vi "About Design.vi"(8 "error in":errorcluster, 10 "Mathcad Output":T1, 11 "DesignRequest":T2) -> (0 "error out":errorcluster)   [LabVIEW 2012, in "Design Server.lvlib"]
uses:
  Design Server.lvlib
  Design Request.ctl
  Variable cluster.ctl
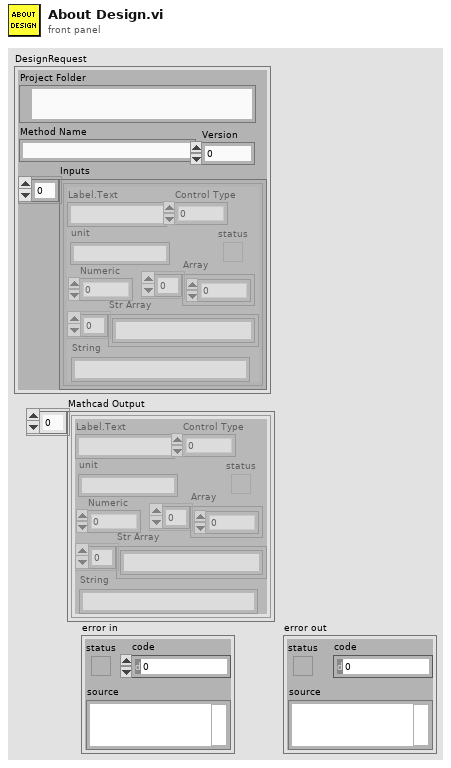
[diagram p1: front panel]
types:
  T1 = typedef "Design Server.lvlib/Variable cluster.ctl" = cluster{"Label.Text":string, "Control Type":u32, "Numeric":dbl, "Array":dbl[], "status":bool, "Str Array":string[], "String":string, "unit":string}[]
  T2 = typedef "Design Server.lvlib/Design Request.ctl" = cluster{"Project Folder":path, "Method Name":string, "Inputs":T1, "Version":i32}
  T3 = enum16{"open", "replace", "create", "open or create", "replace or create", "replace or create with confirmation"}
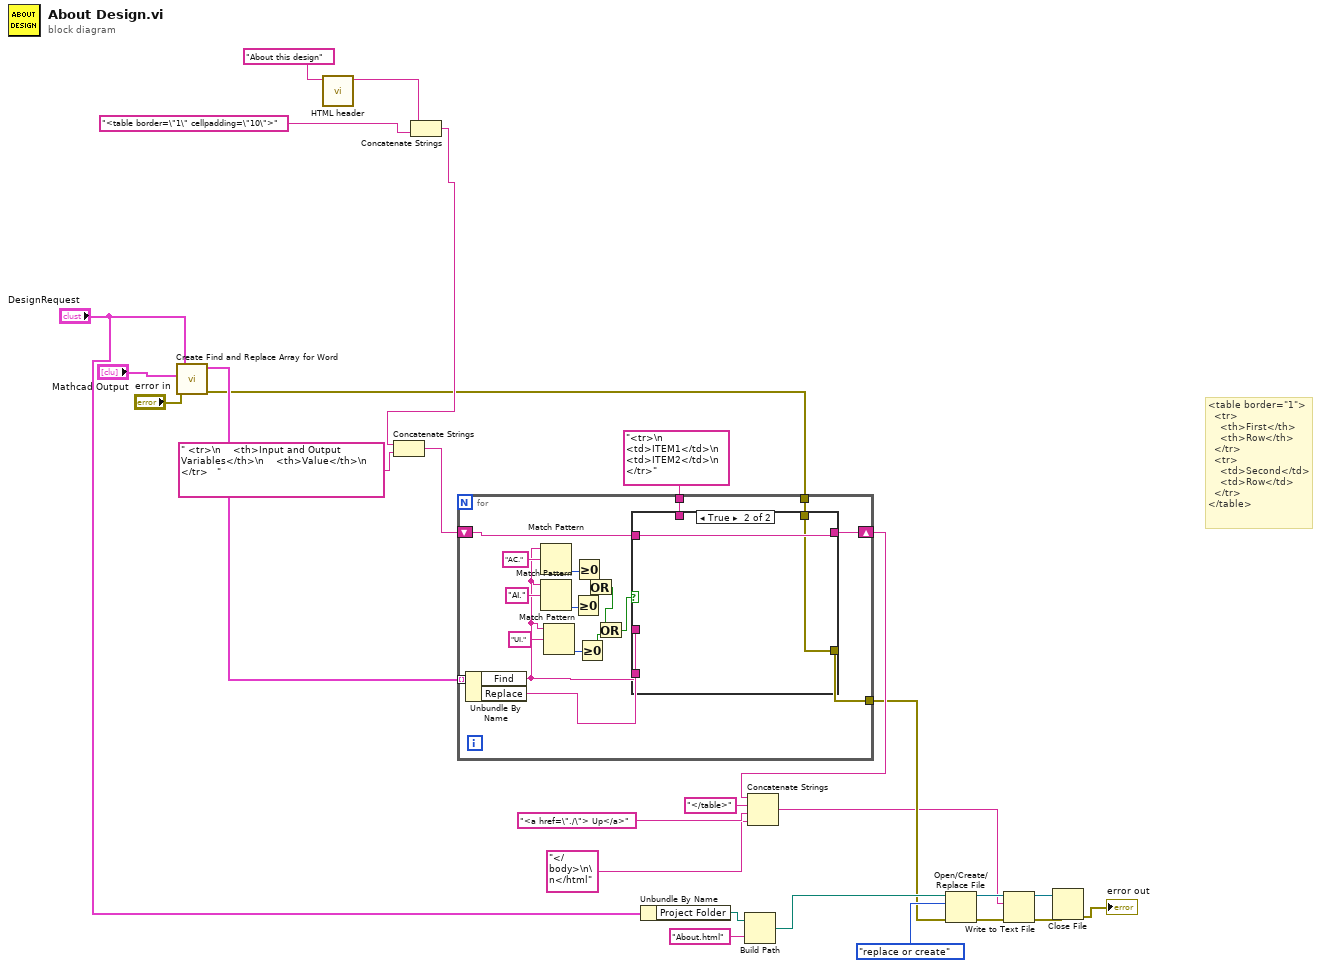
[diagram p0: block diagram]
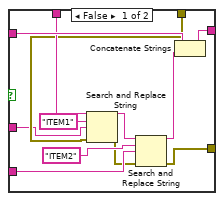
[diagram p2: hidden frame]
diagram:
  # "<table border=\"1\">\n  <tr>\n    <th>First</th>\n    <th>Row</th>\n  </tr>   \n  <tr>\n    <td>Second</td>\n    <td>Row</td>\n  </tr>\n</table>"
  n1 = call "Create Find and Replace Array for Word.vi"("error in"="error in", "Mathcad Output"="Mathcad Output", "DesignRequest"="DesignRequest") -> ("error out"=w1:errorcluster, "Find-Replace"=w17:cluster{"Find":string, "Replace":string}[])  [unwired: 7 in]
  n2 = call "HTML header.vi"("Title"="About this design") -> ("HTML header"=w26:string)  [unwired: 10 in]
  n3 = Concatenate Strings(w26, "<table border=\"1\" cellpadding=\"10\">" ("string")) -> (w3:string)
  n4 = Concatenate Strings(w3, " <tr>\n    <th>Input and Output Variables</th>\n    <th>Value</th>\n  </tr>   " ("string")) -> (w20:string)
  n5 = for {
    tunnel: w17 -> [w46] mode=indexing
    shift-right: [w42] -> w23
    shift-left: w20 -> [w45]
    tunnel: "<tr>\n    <td>ITEM1</td>\n    <td>ITEM2</td>\n  </tr>" -> [w44]
    tunnel: w1 -> [w41]
    tunnel: [w40] -> w9
    n6 = Unbundle By Name(w46) -> ("Find"=w33:string, "Replace"=w43:string)
    n7 = Match Pattern(string=w33, regular expression="AC.") -> (offset past match=w37:i32)  [unwired: 1 in, 3 out]
    n8 = Match Pattern(string=w33, regular expression="AI.") -> (offset past match=w36:i32)  [unwired: 1 in, 3 out]
    n9 = Match Pattern(string=w33, regular expression="UI.") -> (offset past match=w32:i32)  [unwired: 1 in, 3 out]
    n10 = Greater Or Equal To 0?(x=w36) -> (x >= 0?=w31:bool)
    n11 = Greater Or Equal To 0?(x=w37) -> (x >= 0?=w35:bool)
    n12 = Greater Or Equal To 0?(x=w32) -> (x >= 0?=w29:bool)
    n13 = Or(x=w35, y=w31) -> (x .or. y?=w30:bool)
    n14 = Or(x=w30, y=w29) -> (x .or. y?=w28:bool)
    n15 = case shown="True" w28 {
      tunnel: w45 -> [w58 w60]
      tunnel: w44 -> [w57 _]
      tunnel: w43 -> [w53 _]
      tunnel: [w51 w60] -> w42
      tunnel: w41 -> [w50 w59]
      tunnel: [w48 w59] -> w40
      tunnel: w33 -> [w47 _]
      frame False {
        n16 = Search and Replace String(input string=w57, search string="ITEM1", replace string=w47, error in=w50) -> (result string=w56:string, error out=w49:errorcluster)  [unwired: 4 in, 2 out]
        n17 = Search and Replace String(input string=w56, search string="ITEM2", replace string=w53, error in=w49) -> (result string=w52:string, error out=w48:errorcluster)  [unwired: 4 in, 2 out]
        n18 = Concatenate Strings(w58, w52) -> (w51:string)
      }
      frame True {
      }
    }
  }
  n19 = Unbundle By Name("DesignRequest") -> ("Project Folder"=w12:path)
  n20 = Build Path(base path=w12, name or relative path="About.html" ("File Type")) -> (appended path=w13:path)
  n21 = Concatenate Strings(w23, "</table>" ("string"), "<a href=\"./\"> Up</a>" ("string"), "</body>\n\n</html") -> (w7:string)
  n22 = Open/Create/Replace File(file path (use dialog)=w13, error in=w9, operation (0:open)=T3."replace or create") -> (refnum out=w8:refnum<file>, error out=w10:errorcluster)  [unwired: 3 in, 1 out]
  n23 = Write to Text File(file (use dialog)=w8, text=w7, error in=w10) -> (refnum out=w5:refnum<file>, error out=w6:errorcluster)  [unwired: 1 in, 1 out]
  n24 = Close File(refnum=w5, error in=w6) -> (error out=→"error out":errorcluster)  [unwired: 1 out]
